vi "Accuracy.vi"() -> ()   [LabVIEW 2014]
uses:
  Measurement.ctl
  <vilib>/ptbypt/NI_PtbyPt.lvlib
  <vilib>/Analysis/NI_AALBase.lvlib
  <vilib>/National Instruments/Variant Ring Buffer/Ring Buffer.lvclass
panel:
  in  "stop":bool
  in  "True":dbl
  in  "Tab Control":enum32{"Indicators", "Chart"}(tab)
  out "Accurate":T1 {"Mean" format="%.2f"; "Std. Dev." format="%.2f"; "Recent" scale=0.0..100.0}
  out "Inaccurate":T1 {"Mean" format="%.2f"; "Std. Dev." format="%.2f"; "Recent" scale=0.0..100.0}
  out "Precise (repeatable)":T1 {"Mean" format="%.2f"; "Std. Dev." format="%.2f"; "Recent" scale=0.0..100.0}
  out "Lots of digits":T1 {"Mean" format="%.6f"; "Std. Dev." format="%.6f"; "Recent" scale=0.0..100.0 scale format="%_6f"}
  out "Chart 3":T2(graph)
  out "Chart 2":T2(graph)
  out "Chart":T2(graph)
  # "This can be good enough if only measurement differences are important"
  # "\"Precision\" (number of digits shown) is worthless (unless it's also accurate)"
  # "Most often, this is all that matters"
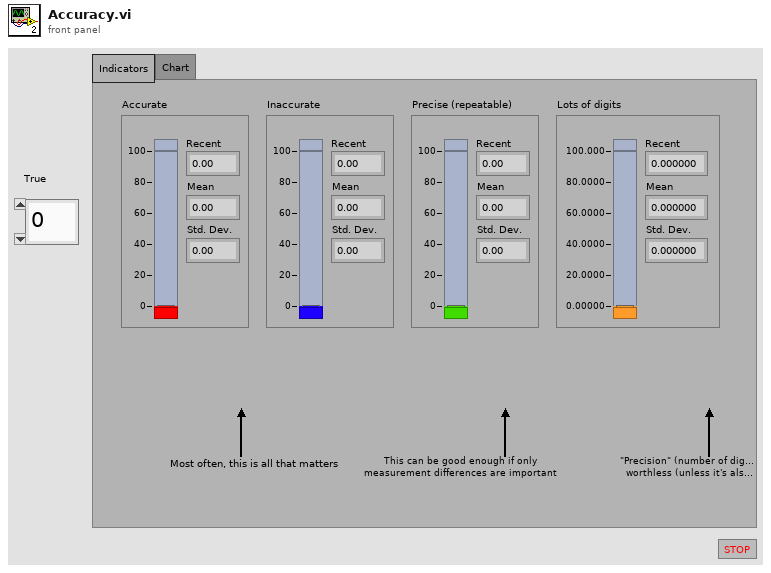
[diagram p1: front panel]
types:
  T1 = typedef "Measurement.ctl" = cluster{"Recent":dbl, "Mean":dbl, "Std. Dev.":dbl}
  T2 = cluster{"standard deviation":dbl, "standard deviation":dbl}
  T3 = cluster{dbl, "mean":dbl, "standard deviation":dbl}
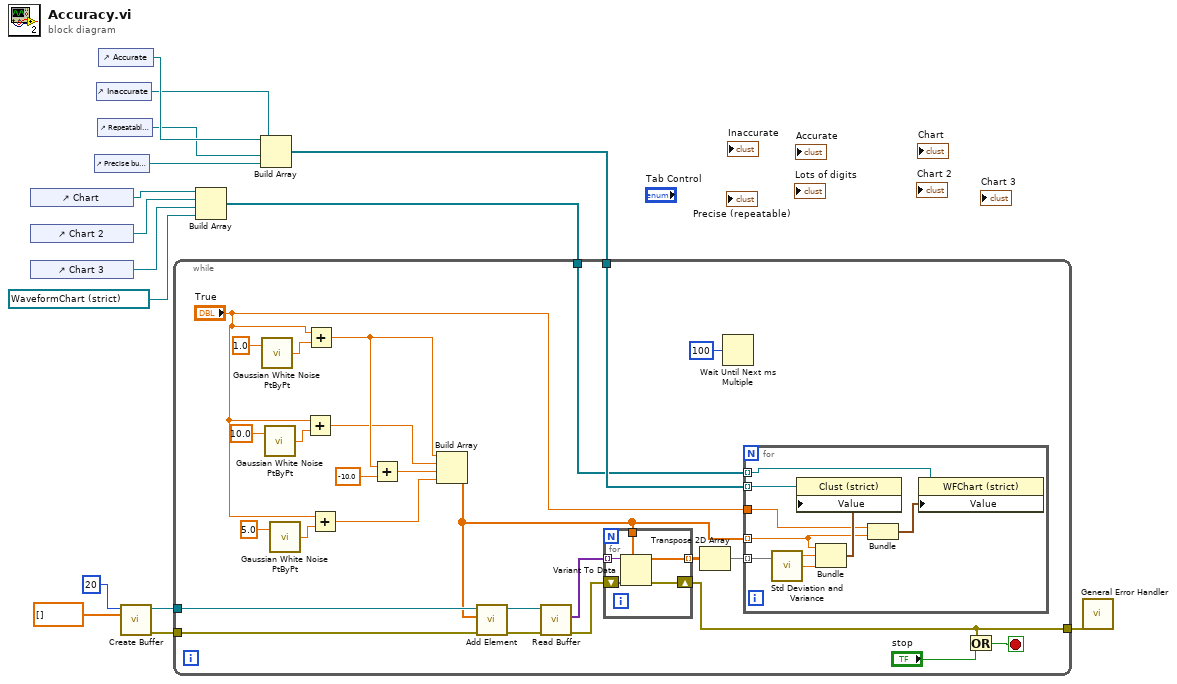
[diagram p0: block diagram]
diagram:
  n1 = control-ref of="Chart"() -> (w5:refnum<vi>)
  n2 = control-ref of="Chart 2"() -> (w4:refnum<vi>)
  n3 = control-ref of="Chart 3"() -> (w3:refnum<vi>)
  n4 = control-ref of="Precise but innaccurate"() -> (w9:refnum<vi>)
  n5 = control-ref of="Inaccurate"() -> (w11:refnum<vi>)
  n6 = control-ref of="Repeatable but inaccurate"() -> (w10:refnum<vi>)
  n7 = control-ref of="Accurate"() -> (w12:refnum<vi>)
  n8 = call <vilib>:"Create Buffer.vi"("Data Type"=dbl[] [] ("appended array"), "Buffer Size"=20) -> ("Error In"=w7:errorcluster, "Ring Buffer Reference"=w13:refnum<data-value>)  [unwired: 8 in]
  n9 = Build Array(w5, w4, w3, refnum<vi> refnum ("element")) -> (w2:refnum<vi>[])
  n10 = Build Array(w12, w11, w10, w9) -> (w8:refnum<vi>[])
  n11 = while {
    tunnel: w13 -> [w31]
    tunnel: w8 -> [w24]
    tunnel: w7 -> [w22]
    tunnel: [w19] -> w6
    tunnel: w2 -> [w18]
    stop <- w20 stop-if-true
    n12 = call <vilib>:"Gaussian White Noise PtByPt.vi"("standard deviation"=1.0) -> ("Gaussian white noise"=w40:dbl)  [unwired: 2 in]
    n13 = call <vilib>:"Gaussian White Noise PtByPt.vi"("standard deviation"=10.0) -> ("Gaussian white noise"=w39:dbl)  [unwired: 2 in]
    n14 = call <vilib>:"Gaussian White Noise PtByPt.vi"("standard deviation"=5.0) -> ("Gaussian white noise"=w37:dbl)  [unwired: 2 in]
    n15 = Add(x="True", y=w39) -> (x+y=w34:dbl)
    n16 = Add(x="True", y=w40) -> (x+y=w35:dbl)
    n17 = Add(x="True", y=w37) -> (x+y=w32:dbl)
    n18 = Add(x=w35, y=-10.0) -> (x+y=w33:dbl)
    n19 = Build Array(w35, w34, w33, w32) -> (w16:dbl[])
    n20 = call <vilib>:"Add Element.vi"("Error In"=w22, "Variant"=w16, "Ring Buffer Reference"=w31) -> ("Error Out"=w29:errorcluster, "Ring Buffer Reference"=w30:refnum<data-value>)  [unwired: 7 in]
    n21 = call <vilib>:"Read Buffer.vi"("Error In"=w29, "Ring Buffer Reference"=w30) -> ("Error Out"=w27:errorcluster, "Array of Variants"=w28:variant[])  [unwired: 7 in, 1 out]
    n22 = for {
      tunnel: w28 -> [w56] mode=indexing
      tunnel: w16 -> [w54]
      shift-right: [w53] -> w19
      shift-left: w27 -> [w55]
      tunnel: [w52] -> w26 mode=indexing
      n23 = Variant To Data(error in=w55, type=w54, Variant=w56) -> (data=w52:dbl[], error out=w53:errorcluster)
    }
    n24 = Transpose 2D Array(2D array=w26) -> (transposed array=w25:dbl[][])
    n25 = Wait Until Next ms Multiple(millisecond multiple=u32 100) -> ()  [unwired: 1 out]
    n26 = for {
      tunnel: w25 -> [w51] mode=indexing
      tunnel: w16 -> [w44] mode=indexing
      tunnel: w24 -> [w50] mode=indexing
      tunnel: w18 -> [w46] mode=indexing
      tunnel: "True" -> [w45]
      n27 = call <vilib>:"Std Deviation and Variance.vi"("X"=w51) -> ("mean"=w48:dbl, "standard deviation"=w49:dbl)  [unwired: 1 in, 1 out]
      n28 = Bundle(w44, "mean"=w48, "standard deviation"=w49) -> (w47:T3)  [unwired: 1 in]
      n29 = property class="Clust (strict)"(reference=w50, "Value"=w47) -> ()  [unwired: 1 in, 2 out]
      n30 = Bundle("True"=w45, w44) -> (w43:cluster{"True":dbl, dbl})  [unwired: 1 in]
      n31 = property class="WFChart (strict)"(reference=w46, "Value"=w43) -> ()  [unwired: 1 in, 2 out]
    }
    n32 = Or(x=w19, y="stop") -> (x .or. y?=w20:bool)
  }
  n33 = call <vilib>:"General Error Handler.vi"("error in (no error)"=w6) -> ()  [unwired: 10 in, 5 out]
